vi "[GV]_GPS Raw_Heading Angle.vi"() -> ()   [LabVIEW 2016]
panel:
  out "GPS Raw_Heading angle":dbl
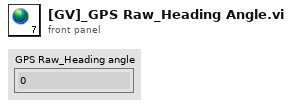
[diagram p1: front panel]
diagram:
